vi "Bury All.vi"(8 "Error In":errorcluster) -> (0 "Error Out":errorcluster)   [LabVIEW 2018, in "Tests.lvlib" / "Bookmark Manager.lvlib" / "Unit.lvlib"]
uses:
  Unit.lvlib
  <vilib>/addons/_JKI Toolkits/Caraya/classes/Test/Test.lvclass
  src/Bookmark Manager/Bookmark Manager.lvlib
  <vilib>/addons/_JKI Toolkits/Caraya/classes/Assert/Assert.lvclass
  src/Toolkit/Toolkit.lvlib
  Tests.lvlib
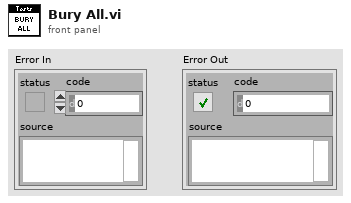
[diagram p1: front panel]
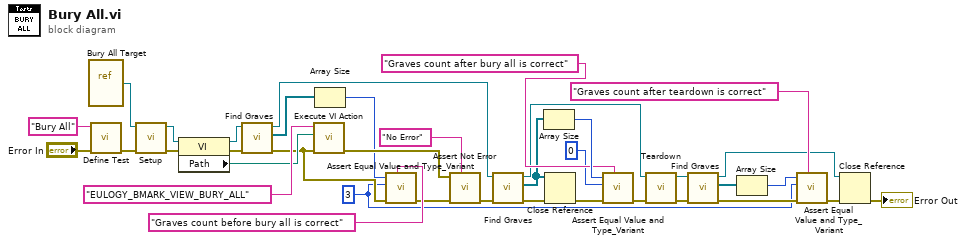
[diagram p0: block diagram]
diagram:
  w1 = 3 ("size(s)")
  n1 = vi-ref "Bury All Target.vi"() -> (w19:refnum<vi>)
  n2 = call <vilib>:"Define Test.vi"("error in (no error)"="Error In", "Label (VI Title)"="Bury All") -> ("error out"=w35:errorcluster)  [unwired: 9 in]
  n3 = call "Setup.vi"("Error In"=w35, "VI In"=w19) -> ("Error Out"=w33:errorcluster, "VI Out"=w32:refnum<vi>)  [unwired: 8 in]
  n4 = property on="Property Node" class="VI"(reference=w32, error in=w33) -> (reference out=w16:refnum<vi>, error out=w17:errorcluster, "Path"=w18:path)
  n5 = call "Find Graves.vi"("Error In"=w17, "VI In"=w16) -> ("Error Out"=w11:errorcluster, "Graves"=w14:refnum<vi>[], "VI Out"=w15:refnum<vi>)  [unwired: 7 in]
  n6 = call "Execute VI Action.vi"("Error In"=w11, "VI"=w18, "Menu Tag"="EULOGY_BMARK_VIEW_BURY_ALL") -> ("Error Out"=w28:errorcluster)  [unwired: 8 in]
  n7 = Array Size(array=w14) -> (size(s)=w13:i32)
  n8 = call <vilib>:"Assert Equal Value and Type_Variant.vi"("Label"="Graves count before bury all is correct", "error in (no error)"=w11, "Y"=w1, "X"=w13) -> ("error out"=w10:errorcluster)  [unwired: 7 in]
  n9 = call <vilib>:"Assert Not Error.vi"("Label"="No Error", "error in (no error)"=w10, "Not Error?"=w28) -> ("error out"=w27:errorcluster)  [unwired: 8 in]
  n10 = call "Find Graves.vi"("Error In"=w27, "VI In"=w15) -> ("Error Out"=w30:errorcluster, "Graves"=w21:refnum<vi>[], "VI Out"=w25:refnum<vi>)  [unwired: 7 in]
  n11 = Array Size(array=w21) -> (size(s)=w31:i32)
  n12 = Close Reference(reference=w21, error in (no error)=w30) -> (error out=w22:errorcluster)
  n13 = call <vilib>:"Assert Equal Value and Type_Variant.vi"("Label"="Graves count after bury all is correct", "error in (no error)"=w22, "Y"=0 ("size(s)"), "X"=w31) -> ("error out"=w26:errorcluster)  [unwired: 7 in]
  n14 = call "Teardown.vi"("Error In"=w26, "VI In"=w25) -> ("Error Out"=w8:errorcluster, "VI Out"=w9:refnum<vi>)  [unwired: 8 in]
  n15 = call "Find Graves.vi"("Error In"=w8, "VI In"=w9) -> ("Error Out"=w7:errorcluster, "Graves"=w4:refnum<vi>[], "VI Out"=w2:refnum<vi>)  [unwired: 7 in]
  n16 = Array Size(array=w4) -> (size(s)=w3:i32)
  n17 = call <vilib>:"Assert Equal Value and Type_Variant.vi"("Label"="Graves count after teardown is correct", "error in (no error)"=w7, "Y"=w1, "X"=w3) -> ("error out"=w5:errorcluster)  [unwired: 7 in]
  n18 = Close Reference(reference=w2, error in (no error)=w5) -> (error out=→"Error Out":errorcluster)
